vi "EletoMatr_1channel.vi"(0 "Input Array X":dbl[][](array[numeric]), 5 "Input data":dbl, 9 "In Row":i32, 11 "In Column":i32, 12 "Input Direction":bool=TRUE) -> (3 "Completed":bool=TRUE, 4 "Out Array X":dbl[][](array[numeric]), 10 "Out Row":i32, 14 "Output Direction":bool=TRUE, 15 "Out Column":i32)   [LabVIEW 2018]
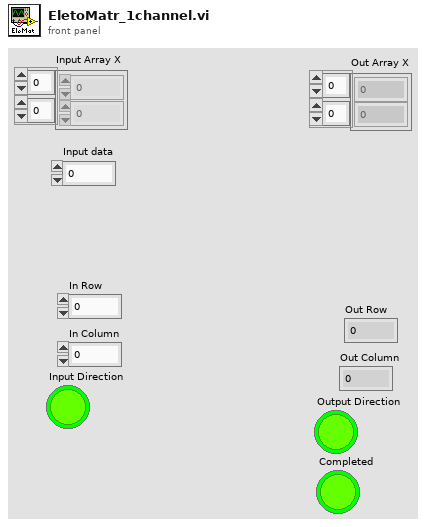
[diagram p1: front panel]
types:
  T1 = typedef "NI_Matrix.lvlib/RealMatrix.ctl" = dbl[][]
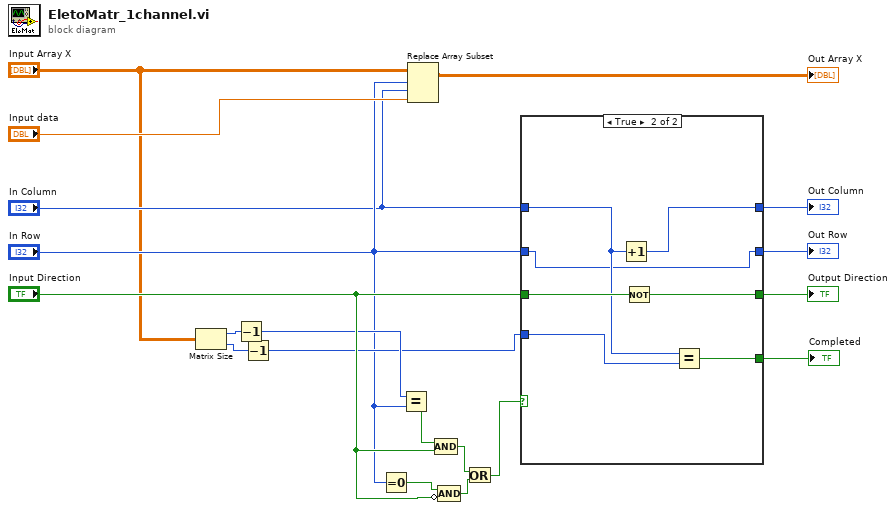
[diagram p0: block diagram]
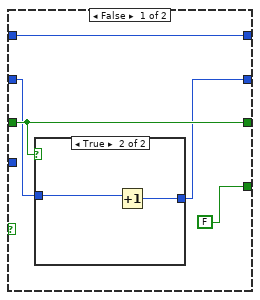
[diagram p2: hidden frame]
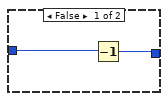
[diagram p3: hidden frame]
diagram:
  n1 = Matrix Size(0:"Input Array X") -> (1:w12:i32, 2:w11:i32)
  n2 = Decrement(x=w12) -> (x-1=w6:i32)
  n3 = Decrement(x=w11) -> (x-1=w5:i32)
  n4 = Equal To 0?(x="In Row") -> (x = 0?=w7:bool)
  n5 = Equal?(x=w6, y="In Row") -> (x = y?=w10:bool)
  n6 = Replace Array Subset(array="Input Array X", new element="Input data", index (row)="In Row", index (col)="In Column") -> (→"Out Array X":T1)
  n7 = Compound Arithmetic op=AND(w10, "Input Direction") -> (w8:bool)
  n8 = Compound Arithmetic op=AND(w7, invert "Input Direction") -> (w14:bool)
  n9 = Or(x=w8, y=w14) -> (x .or. y?=w13:bool)
  n10 = case shown="True" w13 {
    tunnel: "Input Direction" -> [w24 w35]
    tunnel: "In Row" -> [w22 w29]
    tunnel: [w20 w30] -> w18
    tunnel: "In Column" -> [w20 w31]
    tunnel: [w24 w34] -> w17
    tunnel: [w21 w29] -> w16
    tunnel: w5 -> [_ w32]
    tunnel: [FALSE w33] -> w15
    frame False {
      n11 = case shown="True" w24 {
        tunnel: [w26 w28] -> w21
        tunnel: w22 -> [w25 w27]
        frame False {
          n12 = Decrement(x=w25) -> (x-1=w26:i32)
        }
        frame True {
          n13 = Increment(x=w27) -> (x+1=w28:i32)
        }
      }
    }
    frame True {
      n14 = Increment(x=w31) -> (x+1=w30:i32)
      n15 = Not(x=w35) -> (.not. x?=w34:bool)
      n16 = Equal?(x=w31, y=w32) -> (x = y?=w33:bool)
    }
  }
  "Out Row" <- w16
  "Out Column" <- w18
  "Output Direction" <- w17
  "Completed" <- w15
